vi "combineMetrics.vi"(2 "MET Data.csv":path, 3 "ESDU Path":path=path "" caption="start path") -> (0 "ESDU Mean Factors":string[][](array[string]), 1 "Annual Met Data":string[][](array[string]))   [LabVIEW 2018]
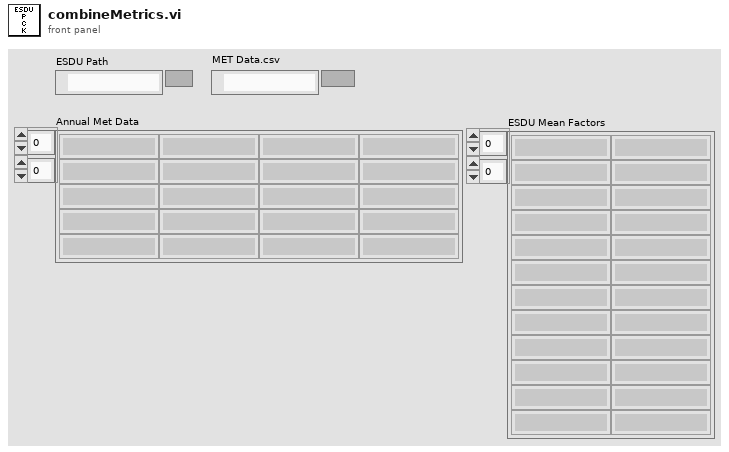
[diagram p1: front panel]
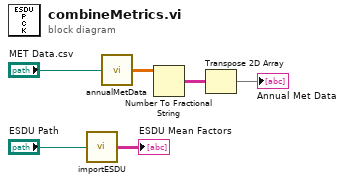
[diagram p0: block diagram]
diagram:
  n1 = call "importESDU.vi"("ESDU Path"="ESDU Path") -> ("ESDU Mean Factors"=→"ESDU Mean Factors":string[][])
  n2 = call "annualMetData.vi"("MET Data.csv"="MET Data.csv") -> ("Annual Met Data"=w5:dbl[][])
  n3 = Number To Fractional String(number=w5) -> (F-format string=w4:string[][])  [unwired: 3 in]
  n4 = Transpose 2D Array(2D array=w4) -> (transposed array=→"Annual Met Data":string[][])
